vi "Update Status Message for Test.vi"(11 "LED Board Power Test in":refnum<class "LED Board Setup.lvclass">) -> ()   [LabVIEW 2015, in "LED Board Setup.lvclass"]
uses:
  LED Board Setup.lvclass
  Test Class/Test Class.lvclass
  Classes/Application/Class/Application.lvclass
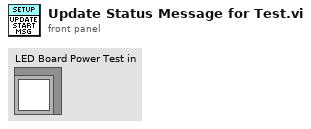
[diagram p1: front panel]
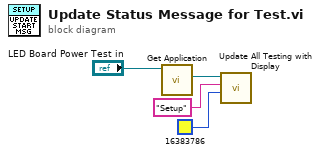
[diagram p0: block diagram]
diagram:
  n1 = call "Get Application.vi"("Test Class in"="LED Board Power Test in") -> ("Application.lvlib:Application.lvclass"=w4:refnum<class "Application.lvclass">)  [unwired: 9 in, 1 out]
  n2 = call "Update All Testing with Display.vi"("BG Color"=u32 16383786, "Message ('')"="Setup", "Application in"=w4) -> ()  [unwired: 7 in, 2 out]
